vi "csv-log-data-headings.vi"(7 "CSV Data Headings":string="timestamp, data1, data2, data3, data4,", 8 "error in (no error)":errorcluster, 9 "keep file open?":bool=TRUE, 11 "Log File Path":path) -> (0 "error out":errorcluster, 2 "Log File Path":path, 3 "Byte Stream File out":refnum<file>)   [LabVIEW 2024]
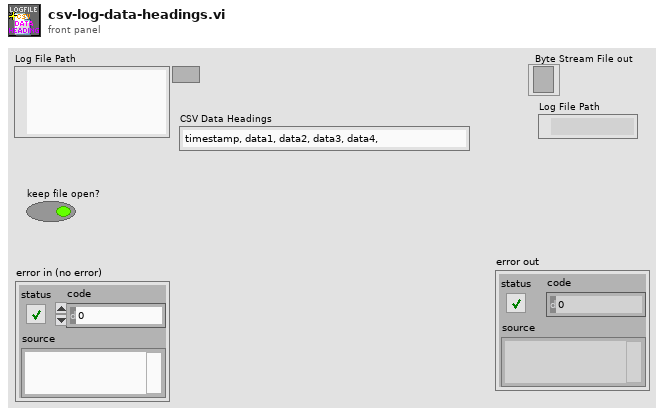
[diagram p1: front panel]
types:
  T1 = enum16{"open", "replace", "create", "open or create", "replace or create", "replace or create with confirmation"}
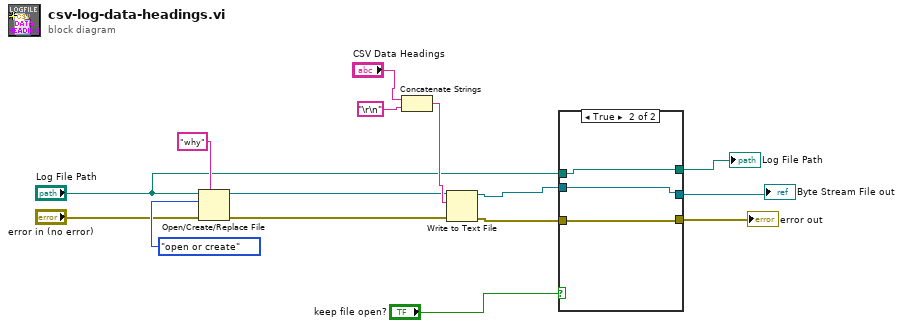
[diagram p0: block diagram]
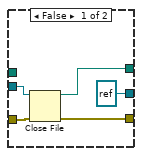
[diagram p2: hidden frame]
diagram:
  n1 = Open/Create/Replace File(file path (use dialog)="Log File Path", error in="error in (no error)", prompt="why", operation (0:open)=T1."open or create") -> (refnum out=w10:refnum<file>, error out=w8:errorcluster)  [unwired: 2 in, 1 out]
  n2 = Concatenate Strings("CSV Data Headings", "\r\n") -> (w13:string)
  n3 = Write to Text File(file (use dialog)=w10, text=w13, error in=w8) -> (refnum out=w4:refnum<file>, error out=w7:errorcluster)  [unwired: 1 in, 1 out]
  n4 = case shown="True" "keep file open?" {
    tunnel: w7 -> [w20 w23]
    tunnel: [w19 w23] -> w6
    tunnel: [refnum<file> refnum ("refnum out") w22] -> w3
    tunnel: "Log File Path" -> [_ w21]
    tunnel: w4 -> [w18 w22]
    tunnel: [w17 w21] -> w1
    frame False {
      n5 = Close File(refnum=w18, error in=w20) -> (path=w17:path, error out=w19:errorcluster)
    }
    frame True {
    }
  }
  "error out" <- w6
  "Byte Stream File out" <- w3
  "Log File Path" <- w1
